vi "HoloPy_test_alloc_CUPY.vi"(7 "Application Directory":path, 8 "error in (no error)":errorcluster, 11 "Refnum in":refnum<k35>) -> (0 "error out":errorcluster, 2 "return value":i32, 3 "Refnum out":refnum<k35>)   [LabVIEW 2023, in "holoPyTracks.lvlib"]
uses:
  holoPyTracks.lvlib
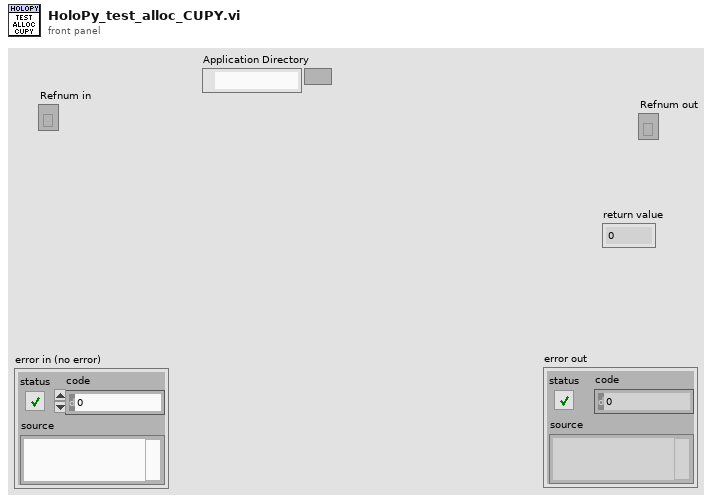
[diagram p1: front panel]
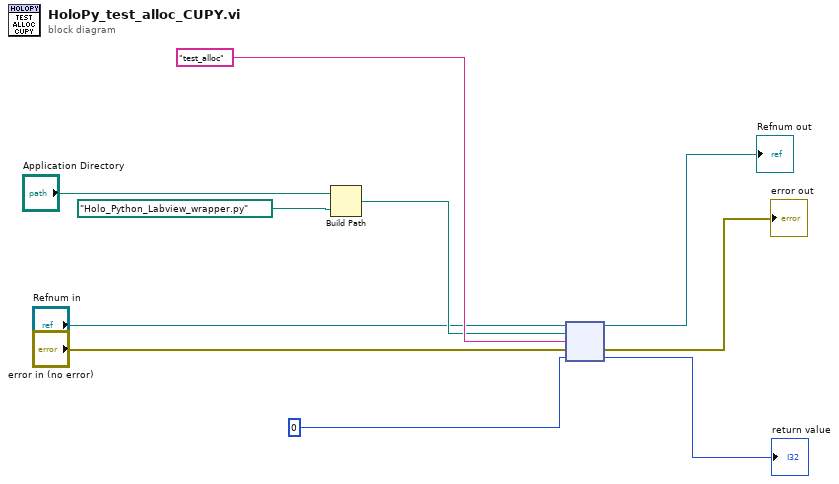
[diagram p0: block diagram]
diagram:
  n1 = Build Path(base path="Application Directory", name or relative path=path "Holo_Python_Labview_wrapper.py") -> (appended path=w9:path)
  n2 = node("Refnum in", w9, "test_alloc" ("function name"), "error in (no error)", 0) -> (→"Refnum out":refnum<k35>, →"error out":errorcluster, →"return value":i32)  [unwired: 2 out]
